vi "SpectrumSubset.vi"(4 "SearchBandMin":dbl, 6 "SearchBandMax":dbl, 10 "Frequencies":dbl[](array[numeric]), 11 "Spectrum":dbl[](array[numeric])) -> (2 "FrequencySubset":dbl[](array[numeric]), 3 "SpectrumSubset":dbl[](array[numeric]))   [LabVIEW 2011]
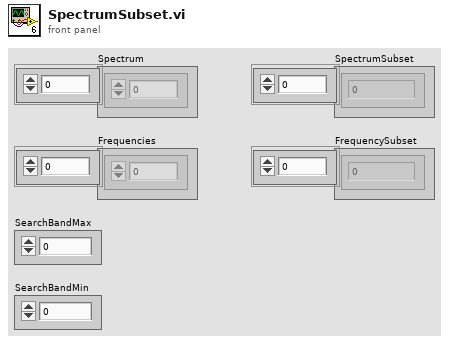
[diagram p1: front panel]
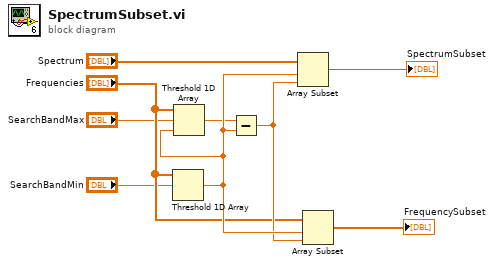
[diagram p0: block diagram]
diagram:
  n1 = Threshold 1D Array(2:"SearchBandMin", 3:"Frequencies") -> (0:w7:dbl)  [unwired: 1 in]
  n2 = Threshold 1D Array(1:w7, 2:"SearchBandMax", 3:"Frequencies") -> (0:w1:dbl)
  n3 = Subtract(x=w1, y=w7) -> (x-y=w6:dbl)
  n4 = Array Subset(array="Spectrum", index=w7, length=w6) -> (→"SpectrumSubset":dbl[])
  n5 = Array Subset(array="Frequencies", index=w7, length=w6) -> (→"FrequencySubset":dbl[])
